vi "lectura imagen modulo vision .vi"() -> ()   [LabVIEW 2020]
panel:
  out "Image":T1(plugin-control)
  in  "Path":path
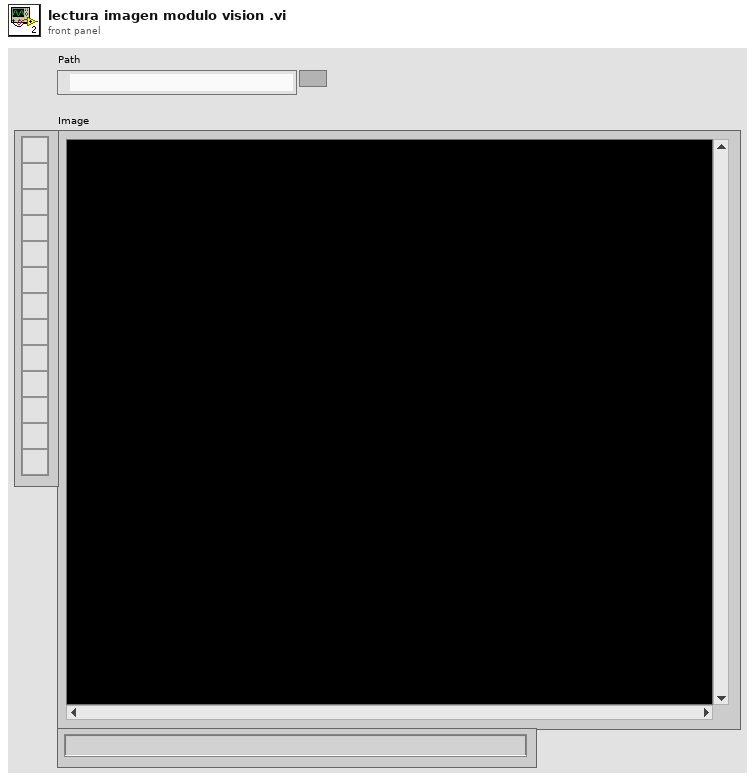
[diagram p1: front panel]
types:
  T1 = typedef "IMAQ Image.ctl" = refnum<image>
  T2 = typedef "Image Type" = u32
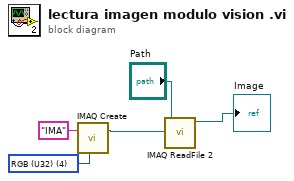
[diagram p0: block diagram]
diagram:
  w3 = T2 4 items=["Grayscale (U8)", "Grayscale (I16)", "Grayscale (SGL)", "Complex (CSG)", "RGB (U32)", "HSL (U32)", "RGB (U64)", "Grayscale (U16)"] ("Image Type")
  n1 = call "IMAQ Create"("Image Name"="IMA", "Image Type"=w3) -> ("New Image"=w2:T1)  [unwired: 3 in, 1 out]
  n2 = call "IMAQ ReadFile 2"("File Path"="Path", "Image"=w2) -> ("Image Out"=→"Image":T1)  [unwired: 5 in, 4 out]
